vi "Clean up BD.vi"(8 "error in (no error)":errorcluster, 11 "VI in":refnum<vi>) -> (0 "error out":errorcluster, 3 "VI out":refnum<vi>)   [LabVIEW 2020, in "Mock Class Generator.lvclass"]
uses:
  Mock Class Generator.lvclass
  <vilib>/Utility/miscctls.llb/LVPointTypeDef.ctl
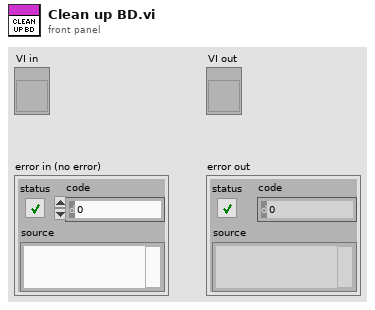
[diagram p1: front panel]
types:
  T1 = typedef "LVPointTypeDef.ctl" = cluster{"Horizontal":i16, "Vertical":i16}
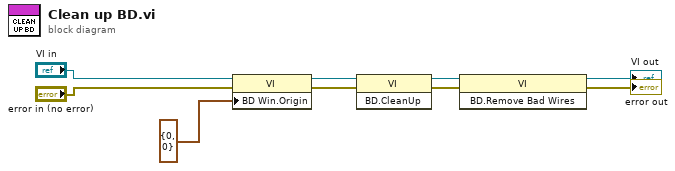
[diagram p0: block diagram]
diagram:
  n1 = property class="VI"(reference="VI in", error in="error in (no error)", "BD Win.Origin"=T1 {"Horizontal"=0, "Vertical"=0} ("Block Diagram Window:Origin")) -> (reference out=w5:refnum<vi>, error out=w6:errorcluster)
  n2 = invoke class="VI" method="BD.CleanUp"(reference=w5, error in=w6) -> (reference out=w2:refnum<vi>, error out=w4:errorcluster)  [unwired: 1 in, 1 out]
  n3 = invoke class="VI" method="BD.Remove Bad Wires"(reference=w2, error in=w4) -> (reference out=→"VI out":refnum<vi>, error out=→"error out":errorcluster)  [unwired: 1 in, 1 out]
